vi "지식인 답변.vi"() -> ()   [LabVIEW 2014]
panel:
  out "웨이브폼 차트":dbl(graph)
  out "array":string[](array[string])
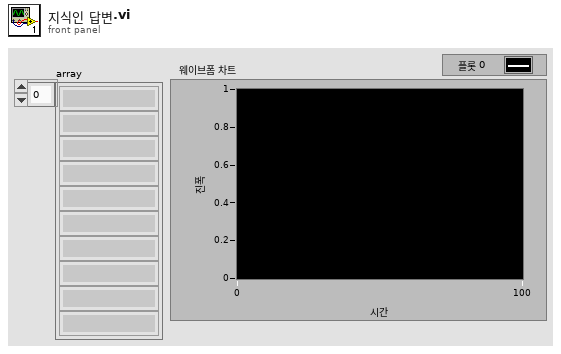
[diagram p1: front panel]
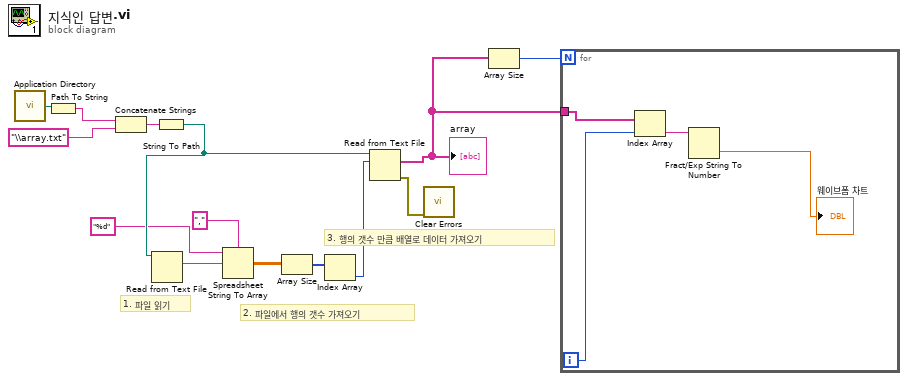
[diagram p0: block diagram]
diagram:
  # "3. 행의 갯수 만큼 배열로 데이터 가져오기"
  # "2. 파일에서 행의 갯수 가져오기"
  # "1. 파일 읽기"
  n1 = call <vilib>:"Application Directory.vi"() -> ("Application Directory"=w3:path)
  n2 = Path To String(path=w3) -> (string=w4:string)
  n3 = Concatenate Strings(w4, "\\array.txt" ("문자열")) -> (w6:string)
  n4 = String To Path(string=w6) -> (path=w12:path)
  n5 = Read from Text File(file (use dialog)=w12) -> (text=w10:string)  [unwired: 1 in, 5 out]
  n6 = Spreadsheet String To Array(delimiter (Tab)=",", format string="%d", spreadsheet string=w10) -> (array=w8:dbl[][])  [unwired: 1 out]
  n7 = Array Size(array=w8) -> (size(s)=w9:i32[])
  n8 = Index Array(array=w9) -> (element=w11:i32)  [unwired: 1 in]
  n9 = Read from Text File(file (use dialog)=w12, count=w11) -> (text=w1:string[], error out=w14:errorcluster)  [unwired: 1 in, 3 out]
  "array" <- w1
  n10 = call <vilib>:"Clear Errors.vi"("error in (no error)"=w14) -> ()  [unwired: 5 in, 2 out]
  n11 = Array Size(array=w1) -> (size(s)=w2:i32)
  n12 = for {
    N: w2 -> [_]
    tunnel: w1 -> [w18]
    i -> [w17]
    n13 = Index Array(array=w18, index=w17) -> (element=w16:string)
    n14 = Fract/Exp String To Number(string=w16) -> (number=→"웨이브폼 차트":dbl)  [unwired: 3 in, 1 out]
  }
